vi "niScope Get Scaling Coefficients.vi"(0 "instrument handle":refnum<k15>, 5 "channels":string="0", 11 "error in":errorcluster) -> (4 "instrument handle out":refnum<k15>, 8 "coefficient info":T1(array[cluster]) {"offset" format="%^_6e"; "gain" format="%^_6e"; "reserved 1" format="%^_6e"; "reserved 2" format="%^_6e"}, 15 "error out":errorcluster)   [LabVIEW 2011]
doc: "Returns coefficients that can be used to scale binary data to volts."
uses:
  niScope_32.dll
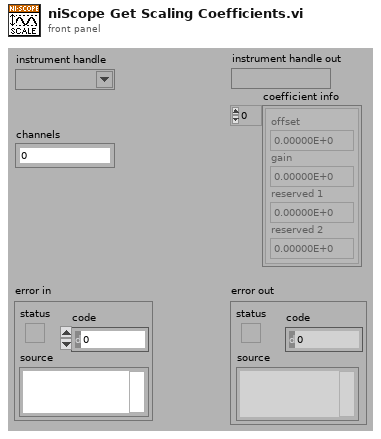
[diagram p1: front panel]
types:
  T1 = cluster{"offset":dbl, "gain":dbl, "reserved 1":dbl, "reserved 2":dbl}[]
  T2 = cluster{"offset":dbl, "gain":dbl, "reserved 1":dbl, "reserved 2":dbl}
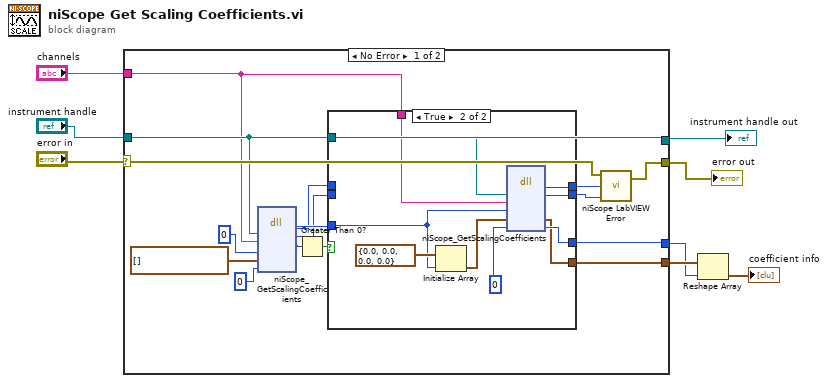
[diagram p0: block diagram]
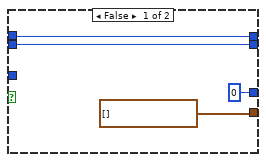
[diagram p2: hidden frame]
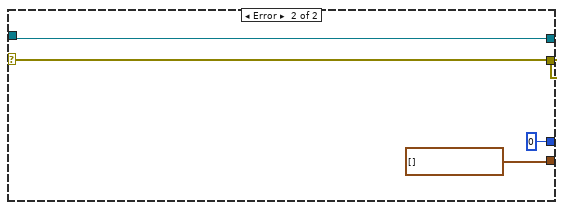
[diagram p3: hidden frame]
diagram:
  n1 = case shown="No Error" "error in" {
    selector: "error in" -> [w20 w39]
    tunnel: [w23 w39] -> w8
    tunnel: "instrument handle" -> [w16 w41]
    tunnel: [w16 w41] -> w7
    tunnel: [w18 T1 [] ("coef info")] -> w3
    tunnel: [w17 0 ("actualSamples")] -> w2
    tunnel: "channels" -> [w15 _]
    frame No Error {
      n2 = dll-call lib="niScope_*.*" fn="niScope_GetScalingCoefficients"("instrument handle"=w16, "channelList"=w15, "arraySize"=0 ("bufferSize"), "coefficientInfo"=T1 [] ("coef info"), "numberOfCoefficientSets"=0 ("numberOfFrequencies")) -> ("status"=w11:i32, "instrument handle"=w10:u32, "numberOfCoefficientSets"=w12:i32)  [unwired: 6 in, 2 out]
      n3 = Greater Than 0?(x=w12) -> (x > 0?=w19:bool)
      n4 = case shown="True" w19 {
        tunnel: [w25 w35] -> w22
        tunnel: [w26 w36] -> w21
        tunnel: w15 -> [_ w30]
        tunnel: w16 -> [_ w31]
        tunnel: w12 -> [_ w29]
        tunnel: [T1 [] ("coef info") w33] -> w18
        tunnel: [0 ("numberOfFrequencies") w34] -> w17
        tunnel: w10 -> [w26 _]
        tunnel: w11 -> [w25 _]
        frame False {
        }
        frame True {
          n5 = Initialize Array(T2 {"offset"=0.0, "gain"=0.0, "reserved 1"=0.0, "reserved 2"=0.0}, w29) -> (w32:T1)
          n6 = dll-call lib="niScope_*.*" fn="niScope_GetScalingCoefficients"("instrument handle"=w31, "channelList"=w30, "arraySize"=w29, "coefficientInfo"=w32, "numberOfCoefficientSets"=0 ("numberOfFrequencies")) -> ("status"=w35:i32, "instrument handle"=w36:u32, "coefficientInfo"=w33:T1, "numberOfCoefficientSets"=w34:i32)  [unwired: 5 in, 2 out]
        }
      }
      n7 = call <instrlib>:"niScope LabVIEW Error.vi"("instrument handle"=w21, "niScope error code (0)"=w22, "error in (no error)"=w20) -> ("error out"=w23:errorcluster)  [unwired: 2 in]
    }
    frame Error {
    }
  }
  "error out" <- w8
  "instrument handle out" <- w7
  n8 = Reshape Array(w3, w2) -> (→"coefficient info":T1)
